vi "Create Servo Motor.vi"(8 "error in (no error)":errorcluster, 9 "apply offset angle from file (T)":bool=TRUE, 10 "servo ID":i32, 11 "starter kit servo motor in":refnum<class "NI_Robotics_Starter Kit Servo Motor.lvclass">) -> (0 "error out":errorcluster, 3 "starter kit servo motor out":refnum<class "NI_Robotics_Starter Kit Servo Motor.lvclass">)   [LabVIEW 2017, in "NI_Robotics_Starter Kit Servo Motor.lvclass"]
uses:
  <vilib>/robotics/Starter Kit/Servo Motor/NI_Robotics_Starter Kit Servo Motor.lvclass
  <vilib>/robotics/Starter Kit/Servo Motor/NI_Robotics_Starter Kit Servo Motor.lvclass/NI_Robotics_Starter Kit Servo Motor.ctl
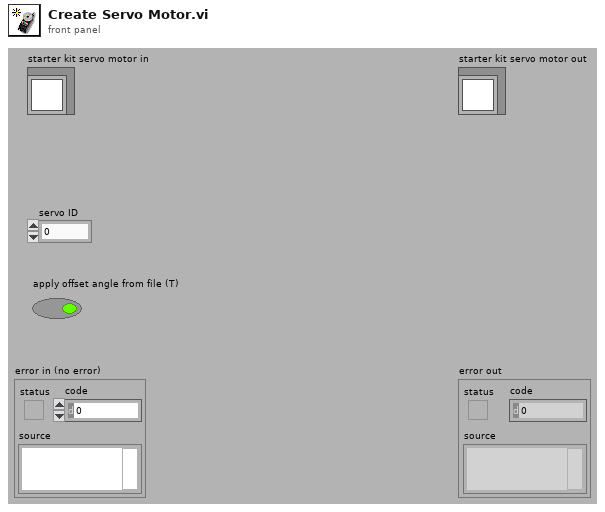
[diagram p1: front panel]
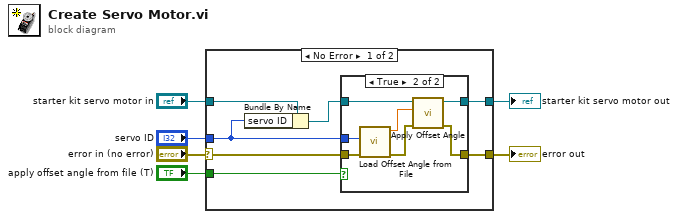
[diagram p0: block diagram]
diagram:
  n1 = case shown="No Error" "error in (no error)" {
    selector: "error in (no error)" -> [w11 w24]
    tunnel: [w10 w24] -> w5
    tunnel: "starter kit servo motor in" -> [w8 w23]
    tunnel: [w12 w23] -> w4
    tunnel: "servo ID" -> [w9 _]
    tunnel: "apply offset angle from file (T)" -> [w7 _]
    frame No Error {
      n2 = Bundle By Name(cluster=w8, "servo ID"=w9) -> (w13:refnum<class "NI_Robotics_Starter Kit Servo Motor.lvclass">)
      n3 = case shown="True" w7 {
        tunnel: w13 -> [w15 w22]
        tunnel: [w15 w21] -> w12
        tunnel: w11 -> [w14 w18]
        tunnel: [w14 w17] -> w10
        tunnel: w9 -> [_ w16]
        frame False {
        }
        frame True {
          n4 = call <vilib>:"Load Offset Angle from File.vi"("error in (no error)"=w18, "servo ID (0)"=w16) -> ("error out"=w19:errorcluster, "ccw offset angle (rad)"=w20:dbl)  [unwired: 7 in, 1 out]
          n5 = call <vilib>:"Apply Offset Angle.vi"("error in (no error)"=w19, "ccw offset angle (rad)"=w20, "servo motor in"=w22) -> ("error out"=w17:errorcluster, "servo motor out"=w21:refnum<class "NI_Robotics_Starter Kit Servo Motor.lvclass">)  [unwired: 7 in]
        }
      }
    }
    frame Error {
    }
  }
  "error out" <- w5
  "starter kit servo motor out" <- w4
